vi "vTab_9234_CHx3.vi"() -> ()   [LabVIEW 2018]
uses:
  <vilib>/Utility/sysdir.llb/System Directory Type.ctl
  <vilib>/measure/mamon.llb/Trigger Detection for 1 Channel.vi
  <vilib>/express/express analysis/Spectral/Block/exnSpectralBlock spectral measurements peak poly.vi
  <vilib>/express/express analysis/Spectral/Block/exnSpectralBlock spectral measurements peak DDT.vi
  <vilib>/ErrorRing/Error Ring.xnode
  <vilib>/express/express analysis/Spectral/XNode/ExpressSpectralMeasurementsBlockNode.xnode
  <vilib>/measure/NI_MAPro.lvlib
  <vilib>/Utility/config.llb/NI_LVConfig.lvlib
panel:
  out "SVING":bool caption="存檔"
  in  "Open Folder":bool
  in  "Enable Saving":bool
  in  "Status":bool
  out "DA":bool caption="觸發"
  out "Time":timestamp format="%<%Y/%m/%d   %H:%M:%S>T"
  in  "Tab Control":enum32{"觸發訊號", "參數設定"}(tab)
  out "TD-P2P-Ch 3":dbl
  out "FFT-P2P-Ch 3":dbl
  out "TD-P2P-Ch 2":dbl
  out "FFT-P2P-Ch 2":dbl
  out "TD-P2P-Ch 1":dbl
  out "FFT-P2P-Ch 1":dbl
  out "CH3-Z-FFT":dynamicdata(graph)
  out "CH2-Y-FFT":dynamicdata(graph)
  out "CH1-X-FFT":dynamicdata(graph)
  out "CH3-Z-Timedomain":dynamicdata(graph)
  out "CH2-Y-Timedomain":dynamicdata(graph)
  out "CH1-X-Timedomain":dynamicdata(graph)
  in  "Lower Cut-Off (Hz)":dbl=100.0
  in  "Pre Samples":i32
  in  "Trigger Level":dbl=0.1 format="%#_13g"
  in  "觸發軸":enum32{"Channel 1", "Channel 2", "Channel 3"}(ring)
  in  "DAQ Device (請選取 NI 9234 )":tag="cDAQ1Mod1"
  in  "ABORT":bool
  in  "Run":bool
  out "DAQ Stoped":bool
  out "DAQ Data":dynamicdata(graph)
  in  "PAUSE":bool
  out "DAQ Error":errorcluster
  out "DAQ (N)":i32
  out "Main (N)":i32
  out "Buffer in Queue":i32(slide) scale=0.0..100.0
  out "Processed":dynamicdata(graph)
  in  "Sample Rate":dbl=10000.0 format="%#_13g"
  in  "Samples to Read":i32=10000
  in  "Trigger Slope":enum16{"Falling Edge", "Rising Edge"}(ring)=enum."Rising Edge"
  # "使用前請至 參數設置 設定"
  # "本頁畫面顯示為 觸發後訊號"
  # "FFT Filter by useing High-pass with Lower Cut-Off (Hz)"
  # "擷取卡設定"
  # "(系統開啟後修改無效)"
  # "軟體觸發設定"
  # "(修改即套用)"
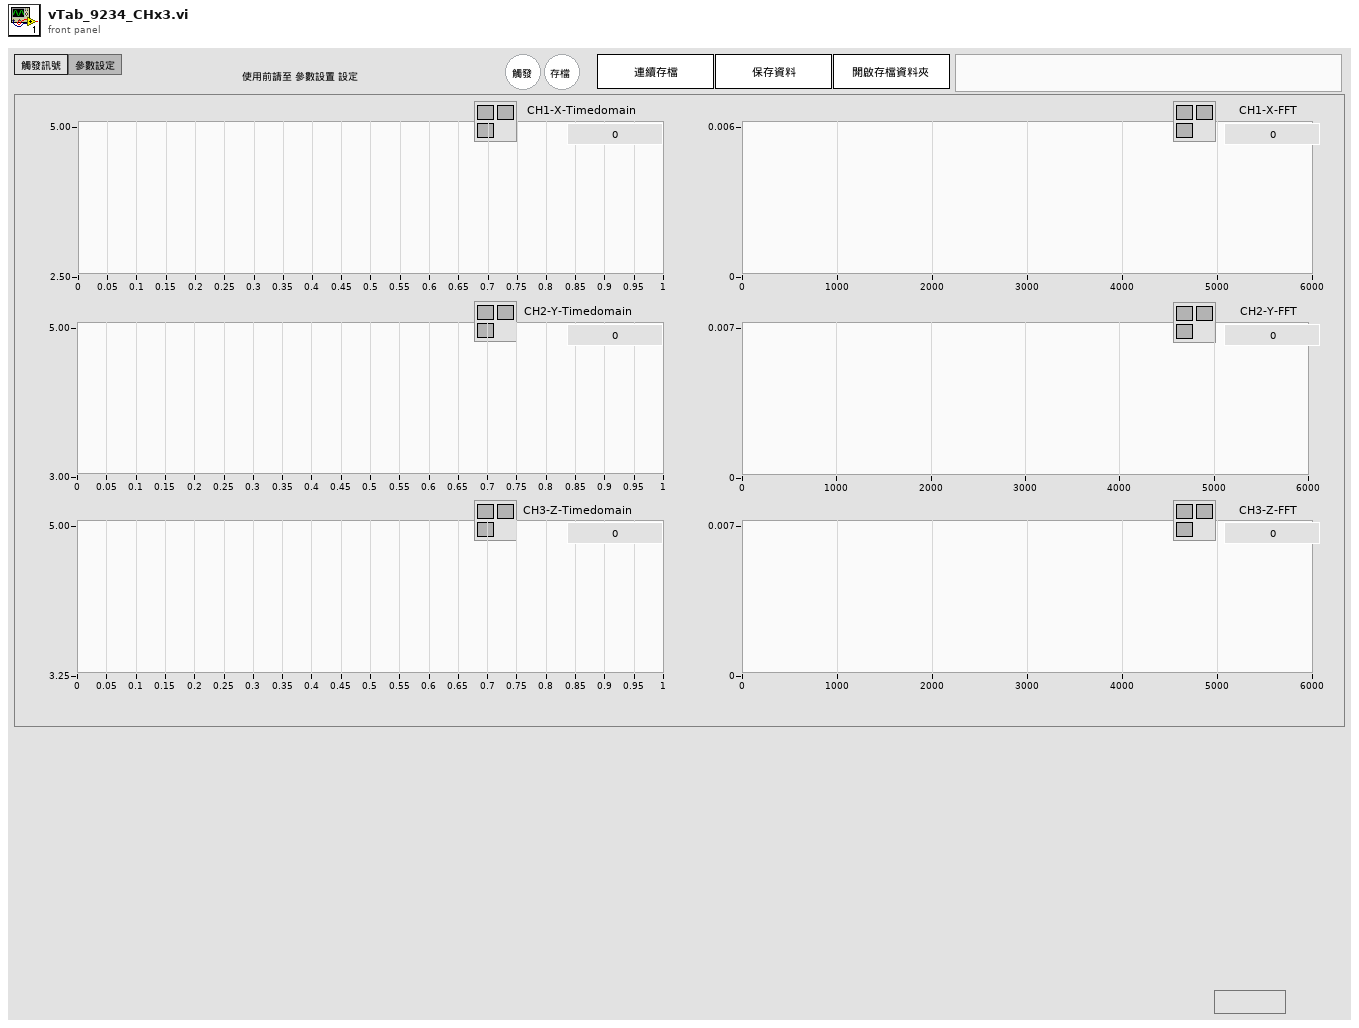
[diagram p1: front panel]
types:
  T1 = typedef "NI_LVConfig.lvlib/Config Data RefNum.ctl" = refnum<k1>
  T2 = enum8{"Enabled", "Disabled", "Disabled and Grayed Out"}
  T3 = cluster{"averaging mode":u16, "weighting mode":u16, "number of averages":u32}
  T4 = cluster{"dB On (F)":bool, "unwrap phase (F)":bool, "convert to degree (F)":bool}
  T5 = typedef "System Directory Type.ctl" = i32
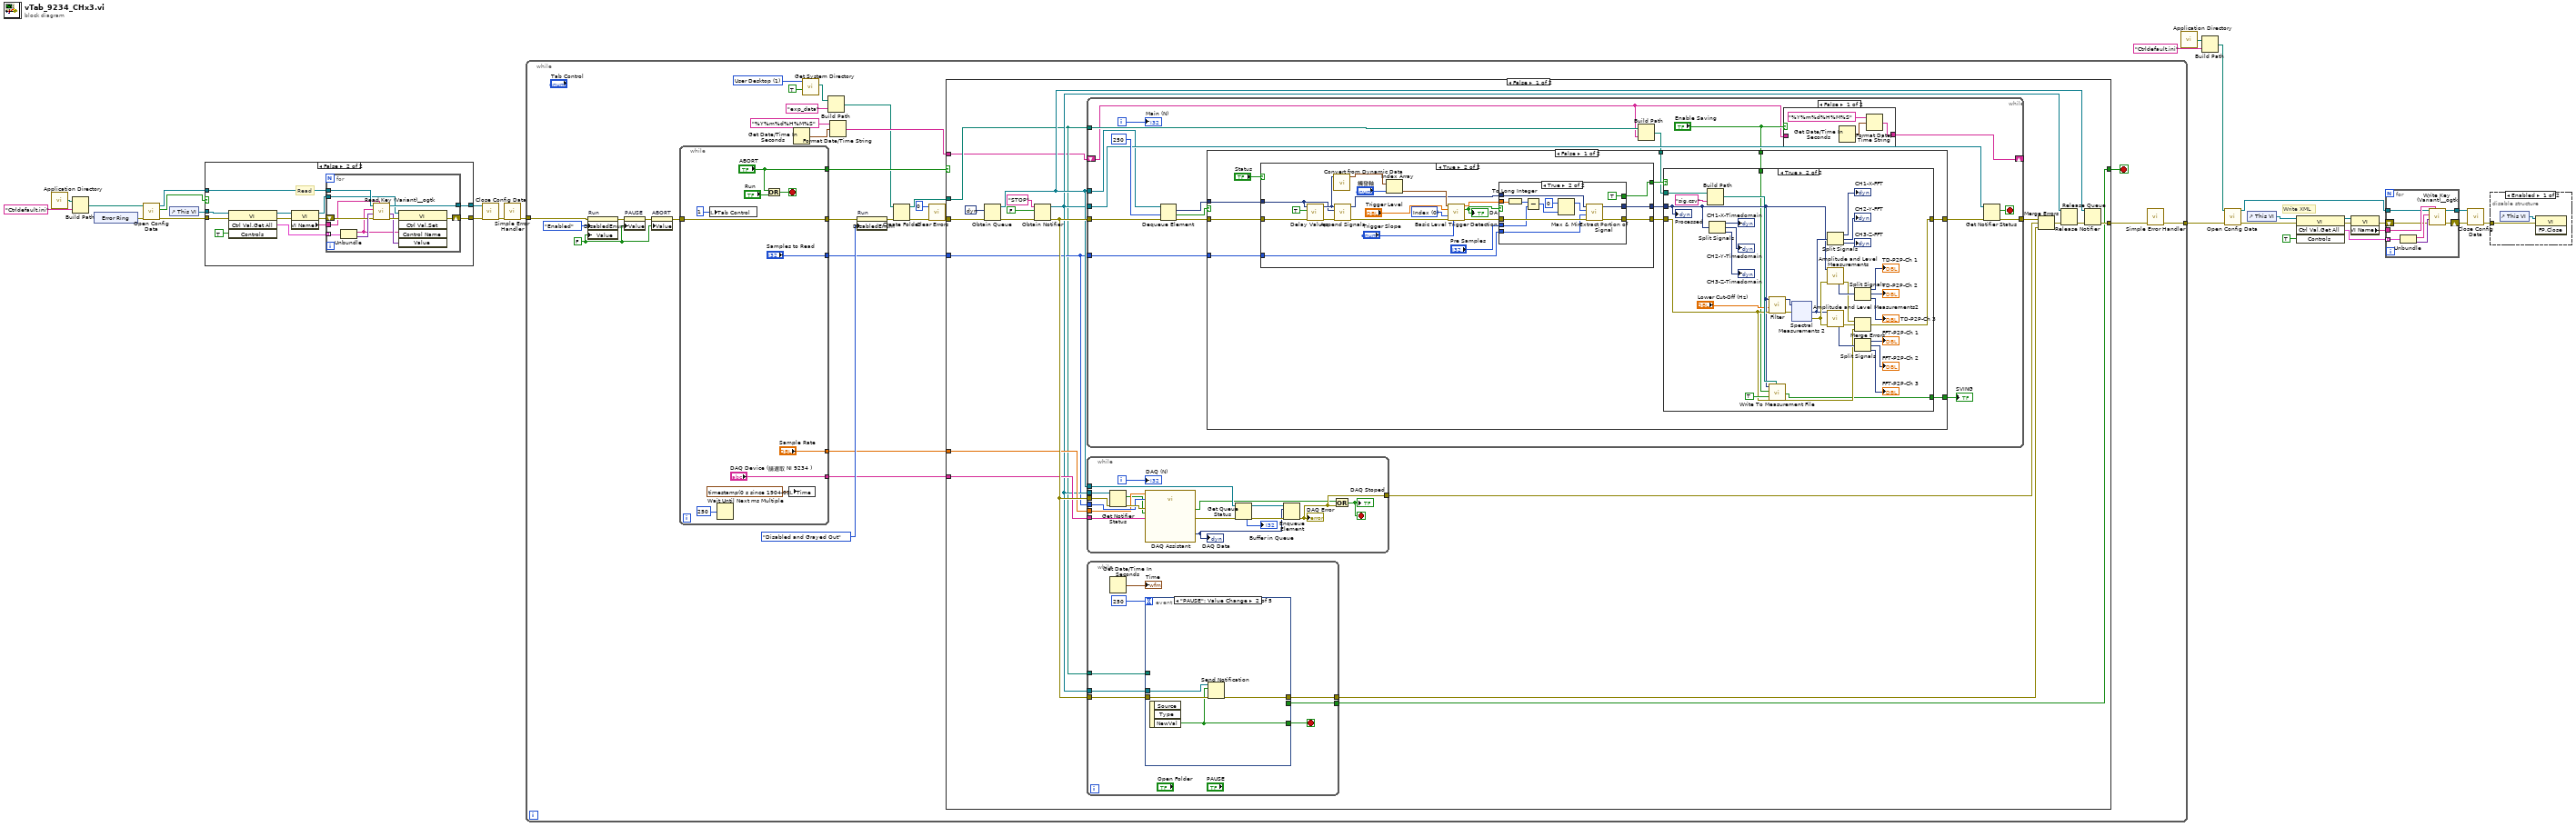
[diagram p0: block diagram]
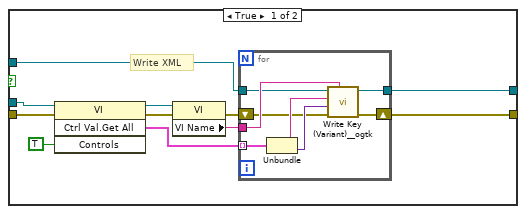
[diagram p2: hidden frame]
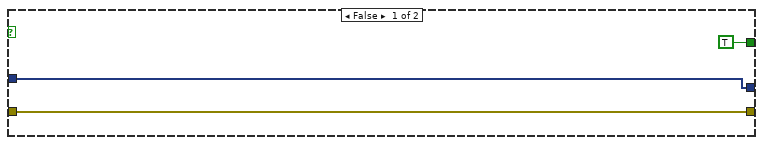
[diagram p5: hidden frame]
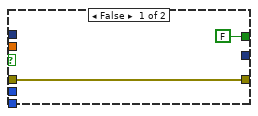
[diagram p6: hidden frame]
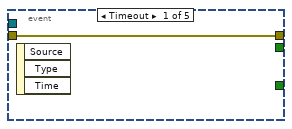
[diagram p9: hidden frame]
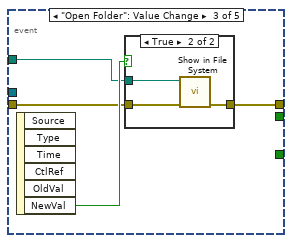
[diagram p10: hidden frame]
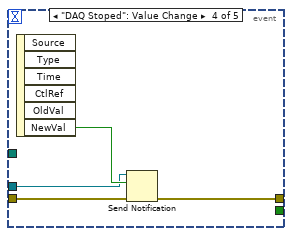
[diagram p12: hidden frame]
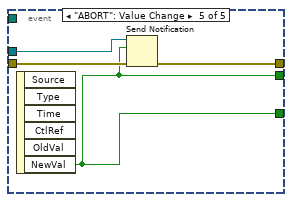
[diagram p13: hidden frame]
diagram:
  # "Write XML"
  n1 = call <vilib>:"Application Directory.vi"() -> ("Application Directory"=w1:path)
  n2 = Build Path(base path=w1, name or relative path="Ctrldefault.ini") -> (appended path=w28:path)
  n3 = xnode "Error Ring"() -> ("error out"=w20:errorcluster)
  n4 = call <vilib>:"Open Config Data.vi"("error in (no error)"=w20, "configuration file path"=w28) -> ("error out"=w25:errorcluster, "file created?"=w21:bool, "refnum"=w18:T1)  [unwired: 7 in]
  n5 = control-ref of="This VI"() -> (w19:refnum<vi>)
  n6 = case shown="False" w21 {
    tunnel: [w33 w53] -> w26
    tunnel: w25 -> [w31 w51]
    tunnel: [w29 w49] -> w24
    tunnel: w19 -> [w32 w52]
    tunnel: w18 -> [w34 w54]
    frame True {
      # "Write XML"
      n7 = invoke class="VI" method="Ctrl Val.Get All"(reference=w32, error in=w31, "Controls"=TRUE) -> (reference out=w38:refnum<vi>, error out=w37:errorcluster, "Get All Control Values Variant"=w39:cluster{"Name":string, "Variant Data":variant}[])  [unwired: 1 in, 1 out]
      n8 = property class="VI"(reference=w38, error in=w37) -> (error out=w30:errorcluster, "VI Name"=w36:string)  [unwired: 1 out]
      n9 = for {
        tunnel: w39 -> [w47] mode=indexing
        tunnel: w36 -> [w46]
        tunnel: w34 -> [w44]
        shift-right: [w43] -> w33
        shift-left: w30 -> [w41]
        tunnel: [w40] -> w29
        n10 = Unbundle(w47) -> ("Name"=w45:string, "Variant Data"=w42:variant)
        n11 = call <userlib>:"Write Key (Variant)__ogtk.vi"("section"=w46, "error in (no error)"=w41, "key-value"=w42, "key (optional)"=w45, "refnum"=w44) -> ("error out"=w43:errorcluster, "refnum out"=w40:T1)  [unwired: 5 in]
      }
    }
    frame False {
      # "Read"
      n12 = invoke class="VI" method="Ctrl Val.Get All"(reference=w52, error in=w51, "Controls"=TRUE) -> (reference out=w58:refnum<vi>, error out=w57:errorcluster, "Get All Control Values Variant"=w59:cluster{"Name":string, "Variant Data":variant}[])  [unwired: 1 in, 1 out]
      n13 = property class="VI"(reference=w58, error in=w57) -> (reference out=w48:refnum<vi>, error out=w50:errorcluster, "VI Name"=w56:string)
      n14 = for {
        tunnel: w59 -> [w70] mode=indexing
        tunnel: w56 -> [w63]
        tunnel: w54 -> [w69]
        shift-right: [w64] -> w53
        shift-left: w50 -> [w67]
        tunnel: [w66] -> w49
        tunnel: w48 -> [w62]
        n15 = Unbundle(w70) -> ("Name"=w60:string, "Variant Data"=w68:variant)
        n16 = call <userlib>:"Read Key (Variant)__ogtk.vi"("section"=w63, "error in (no error)"=w67, "type"=w68, "key (optional)"=w60, "refnum"=w69) -> ("error out"=w65:errorcluster, "key-value"=w61:variant, "refnum out"=w66:T1)  [unwired: 3 in, 1 out]
        n17 = invoke class="VI" method="Ctrl Val.Set"(reference=w62, error in=w65, "Control Name"=w60, "Value"=w61) -> (error out=w64:errorcluster)  [unwired: 1 in, 4 out]
      }
    }
  }
  n18 = call <vilib>:"Close Config Data.vi"("error in (no error)"=w26, "refnum"=w24) -> ("error out"=w23:errorcluster)  [unwired: 8 in, 1 out]
  n19 = call <vilib>:"Simple Error Handler.vi"("error in (no error)"=w23) -> ("error out"=w22:errorcluster)  [unwired: 4 in, 4 out]
  n20 = while {
    tunnel: [w98] -> w4
    tunnel: w22 -> [w76]
    stop <- w79 stop-if-true
    w87 = T5 1 items=["User Home"=0, "User Desktop"=1, "User Documents"=2, "User Application Data"=3, "User Preferences"=4, "User Temporary"=5, "Public Documents"=6, "Public Application Data"=7, "Public Preferences"=8, "Public Cache"=13, "System Core Libraries"=9, "System Installed Libraries"=10, "Application Files"=11, "Boot Volume Root"=12] ("system directory type")
    w92 = FALSE ("stop 3")
    n21 = property on="Run" class="Bool (strict)"(error in=w76, "DisabledEnum"=T2."Enabled" ("Disabled"), "Value"=w92) -> (error out=w95:errorcluster)  [unwired: 1 in, 1 out]
    n22 = property on="PAUSE" class="Bool (strict)"(error in=w95, "Value"=w92) -> (error out=w94:errorcluster)  [unwired: 1 in, 1 out]
    n23 = property on="ABORT" class="Bool (strict)"(error in=w94, "Value"=w92) -> (error out=w93:errorcluster)  [unwired: 1 in, 1 out]
    n24 = while {
      tunnel: [w290] -> w75
      tunnel: w93 -> [w290]
      tunnel: ["Samples to Read"] -> w78
      tunnel: ["Sample Rate"] -> w82
      tunnel: ["DAQ Device (請選取 NI 9234 )"] -> w80
      tunnel: ["ABORT"] -> w74
      stop <- w283 stop-if-true
      n25 = local write "Tab Control"(1) -> ()
      n26 = Wait Until Next ms Multiple(millisecond multiple=u32 250) -> ()  [unwired: 1 out]
      n27 = Or(x="ABORT", y="Run") -> (x .or. y?=w283:bool)
      n28 = local write "Time"(timestamp(0 s since 1904-01-01) ("Time 2")) -> ()
    }
    n29 = Get Date/Time In Seconds() -> (seconds since 1Jan1904=w73:timestamp)
    n30 = call <vilib>:"Get System Directory.vi"("create directory if not found? (F)"=TRUE, "system directory type"=w87) -> ("system directory"=w89:path)  [unwired: 9 in]
    n31 = Build Path(base path=w89, name or relative path="exp_data") -> (appended path=w71:path)
    n32 = Format Date/Time String(time format string (%c)="%Y%m%d%H%M%S", seconds (now)=w73) -> (date/time string=w72:string)  [unwired: 1 in]
    n33 = property on="Run" class="Bool (strict)"(error in=w75, "DisabledEnum"=T2."Disabled and Grayed Out" ("Disabled")) -> (error out=w90:errorcluster)  [unwired: 1 in, 1 out]
    n34 = Create Folder(path (use dialog)=w71, error in=w90) -> (created path=w77:path, error out=w84:errorcluster)  [unwired: 1 in, 1 out]
    n35 = call <vilib>:"Clear Errors.vi"("error in (no error)"=w84, "specific error code to clear (0: all)"=0) -> ("error out"=w83:errorcluster)  [unwired: 4 in, 1 out]
    n36 = case shown="False" w74 {
      selector: w74 -> [_ w279]
      tunnel: w83 -> [w111 w280]
      tunnel: w82 -> [w110 _]
      tunnel: [w107 w280] -> w81
      tunnel: w80 -> [w104 _]
      tunnel: [w102 w279] -> w79
      tunnel: w78 -> [w101 _]
      tunnel: w77 -> [w100 _]
      tunnel: w72 -> [w99 _]
      frame False {
        n37 = Obtain Queue(element data type=dynamicdata [] ("data"), error in (no error)=w111) -> (queue out=w109:refnum<queue>, error out=w114:errorcluster)  [unwired: 3 in, 1 out]
        n38 = Obtain Notifier(name (unnamed)="STOP", notification data type=FALSE, error in (no error)=w114) -> (notifier out=w103:refnum<notifier>, error out=w117:errorcluster)  [unwired: 1 in, 1 out]
        n39 = while {
          tunnel: w109 -> [w127]
          tunnel: w117 -> [w134]
          tunnel: [w130] -> w105
          tunnel: w103 -> [w128]
          tunnel: w101 -> [w125]
          tunnel: w100 -> [w123]
          shift-right: [w120] -> _
          shift-left: w99 -> [w119]
          i -> [w136]
          stop <- w129 stop-if-true
          n40 = Dequeue Element(queue=w127, timeout in ms (-1)=250, error in (no error)=w134) -> (element=w133:dynamicdata, timed out?=w126:bool, error out=w132:errorcluster)  [unwired: 1 out]
          n41 = Build Path(base path=w123, name or relative path=w119) -> (appended path=w122:path)
          n42 = case shown="False" w126 {
            tunnel: w133 -> [w150 _]
            tunnel: w132 -> [w148 w232]
            tunnel: [w151 w232] -> w131
            tunnel: w125 -> [w144 _]
            tunnel: w122 -> [w143 _]
            tunnel: [w142 _] -> w124
            tunnel: "Enable Saving" -> [w141 _]
            frame False {
              n43 = case shown="True" "Status" {
                tunnel: [TRUE ("Data Available") w159] -> w145
                tunnel: w150 -> [w154 w164]
                tunnel: [w154 w157] -> w149
                tunnel: w148 -> [w153 w166]
                tunnel: [w153 w158] -> w147
                tunnel: w144 -> [_ w155]
                frame False {
                }
                frame True {
                  w171 = u16 0 items=["Index", "Time"] ("location mode")
                  n44 = call "Delay Values"("error in (no error)"=w166, "Enable"=TRUE, "Signals"=w164) -> ("error out"=w163:errorcluster, "Delayed Signals"=w165:dynamicdata)  [unwired: 7 in]
                  n45 = call "Convert from Dynamic Data"("Dynamic Data Type"=w165) -> ("Array of Waveform"=w175:waveform(dbl)[])  [unwired: 3 in]
                  n46 = call "Append Signals"("error in (no error)"=w163, "Input Signal B"=w164, "Input Signal A"=w165) -> ("error out"=w162:errorcluster, "Appended Signals"=w160:dynamicdata)  [unwired: 7 in]
                  n47 = Index Array(array=w175, index="觸發軸") -> (element=w174:waveform(dbl))
                  n48 = call-poly <vilib>:"Basic Level Trigger Detection.vi"("signal in"=w174, "level"="Trigger Level", "location mode"=w171, "error in (no error)"=w162, "trigger slope"="Trigger Slope") -> ("trigger location"=w168:dbl, "trigger detected?"=w169:bool, "error out"=w161:errorcluster)  [unwired: 8 in]
                  "DA" <- w169
                  n49 = case shown="True" w169 {
                    tunnel: w168 -> [_ w188]
                    tunnel: w161 -> [w176 w189]
                    tunnel: w160 -> [_ w183]
                    tunnel: [FALSE ("Enable") TRUE ("Enable")] -> w159
                    tunnel: [w176 w186] -> w158
                    tunnel: [_ w184] -> w157
                    tunnel: "Pre Samples" -> [_ w181]
                    tunnel: w155 -> [_ w178]
                    frame False {
                    }
                    frame True {
                      n50 = To Long Integer(number=w188) -> (32bit integer=w187:i32)
                      n51 = Subtract(x=w187, y=w181) -> (x-y=w182:i32)
                      n52 = Max & Min(x=0, y=w182) -> (max(x,y)=w179:i32)  [unwired: 1 out]
                      n53 = call "Extract Portion of Signal"("error in (no error)"=w189, "Samples"=w178, "Begin Sample"=w179, "Signals"=w183) -> ("error out"=w186:errorcluster, "Section"=w184:dynamicdata)  [unwired: 6 in]
                    }
                  }
                }
              }
              n54 = case shown="True" w145 {
                tunnel: w149 -> [_ w195]
                tunnel: w147 -> [w190 w197]
                tunnel: [w190 w203] -> w151
                tunnel: w143 -> [_ w201]
                tunnel: [_ w192] -> w142
                tunnel: w141 -> [_ w191]
                frame False {
                }
                frame True {
                  n55 = Build Path(base path=w201, name or relative path="sig.csv") -> (appended path=w199:path)
                  n56 = Split Signals(w195) -> (→"CH1-X-Timedomain":dynamicdata, →"CH2-Y-Timedomain":dynamicdata, →"CH3-Z-Timedomain":dynamicdata)  [unwired: 3 in]
                  n57 = call "Filter"("error in (no error)"=w197, "Lower Cut-Off"="Lower Cut-Off (Hz)", "Signal"=w195) -> ("error out"=w196:errorcluster, "Filtered Signal"=w194:dynamicdata)  [unwired: 7 in]
                  n58 = call "Write To Measurement File"("Signals"=w195, "Enable"=w191, "new_file"=TRUE, "error in (no error)"=w197, "Filename"=w199) -> ("Saving Data"=w192:bool, "error out"=w206:errorcluster)  [unwired: 12 in, 1 out]
                  n59 = xnode ("Spectral Measurements 2")("Signals"=w194, "error in (no error)"=w196) -> ("FFT - (Peak)"=w198:dynamicdata, "error out"=w221:errorcluster)  [unwired: 1 out]
                  n60 = Split Signals(w198) -> (→"CH1-X-FFT":dynamicdata, →"CH2-Y-FFT":dynamicdata, →"CH3-Z-FFT":dynamicdata)  [unwired: 3 in]
                  n61 = call "Amplitude and Level Measurements"("Signals"=w195, "error in (no error)"=w221) -> ("Peak to Peak"=w208:dynamicdata, "error out"=w204:errorcluster)  [unwired: 12 out]
                  n62 = call "Amplitude and Level Measurements2"("Signals"=w198, "error in (no error)"=w221) -> ("Peak to Peak"=w207:dynamicdata, "error out"=w205:errorcluster)  [unwired: 12 out]
                  n63 = Split Signals(w208) -> (→"TD-P2P-Ch 1":dynamicdata, →"TD-P2P-Ch 2":dynamicdata, →"TD-P2P-Ch 3":dynamicdata)  [unwired: 3 in]
                  n64 = Merge Errors(w204, w205, w206) -> (w203:errorcluster)
                  n65 = Split Signals(w207) -> (→"FFT-P2P-Ch 1":dynamicdata, →"FFT-P2P-Ch 2":dynamicdata, →"FFT-P2P-Ch 3":dynamicdata)  [unwired: 3 in]
                  "Processed" <- w195
                }
              }
            }
            frame True {
            }
          }
          "SVING" <- w124
          n66 = case shown="False" "Enable Saving" {
            tunnel: [w137 w140] -> w120
            tunnel: w119 -> [_ w140]
            frame False {
              n67 = Get Date/Time In Seconds() -> (seconds since 1Jan1904=w138:timestamp)
              n68 = Format Date/Time String(time format string (%c)="%Y%m%d%H%M%S", seconds (now)=w138) -> (date/time string=w137:string)  [unwired: 1 in]
            }
            frame True {
            }
          }
          n69 = Get Notifier Status(notifier=w128, error in (no error)=w131) -> (current notification=w129:bool, error out=w130:errorcluster)  [unwired: 3 out]
          "Main (N)" <- w136
        }
        n70 = while {
          tunnel: w109 -> [w247]
          tunnel: [w239] -> w116
          tunnel: w117 -> [w243]
          tunnel: w103 -> [w241]
          tunnel: w101 -> [w238]
          tunnel: w110 -> [w237]
          tunnel: w104 -> [w233]
          i -> [w249]
          stop <- w240 stop-if-true
          n71 = Get Notifier Status(notifier=w241, error in (no error)=w243) -> (current notification=w236:bool, error out=w242:errorcluster)  [unwired: 3 out]
          n72 = call "DAQ Assistant"("rate"=w237, "number of samples"=w238, "error in"=w242, "stop (F)"=w236, "device name"=w233) -> ("data"=w234:dynamicdata, "stopped"=w235:bool, "error out"=w244:errorcluster)  [unwired: 11 in, 1 out]
          "DAQ Data" <- w234
          n73 = Get Queue Status(queue=w247, error in (no error)=w244) -> (queue out=w246:refnum<queue>, error out=w245:errorcluster, # elements in queue=→"Buffer in Queue":i32)  [unwired: 1 in, 5 out]
          n74 = Enqueue Element(queue=w246, element=w234, error in (no error)=w245) -> (error out=w239:errorcluster)  [unwired: 1 in, 2 out]
          "DAQ Error" <- w239
          n75 = Compound Arithmetic op=OR(w235, w239) -> (w240:bool)
          "DAQ Stoped" <- w240
          "DAQ (N)" <- w249
        }
        n76 = while {
          tunnel: w117 -> [w257]
          tunnel: [w256] -> w118
          tunnel: w103 -> [w254]
          tunnel: [w251] -> w102
          tunnel: w100 -> [w250]
          stop <- w252 stop-if-true
          n77 = Get Date/Time In Seconds() -> (seconds since 1Jan1904=→"Time":timestamp)
          n78 = event shown="[1] \"PAUSE\": Value Change" {
            selector: _ -> [_ _ _ _ _]
            dyn-events: _ -> [_ _ _ _ _]
            timeout: 250 -> [_ _ _ _ _]
            tunnel: w257 -> [w258 w262 w265 w274 w278]
            tunnel: [w258 w261 w263 w271 w277] -> w256
            tunnel: w254 -> [_ w260 _ w272 w276]
            tunnel: [_ w259 _ _ w275] -> w252
            tunnel: [_ _ _ _ w275] -> w251
            tunnel: w250 -> [_ _ w264 _ _]
            event Timeout {
              n79 = event-data() -> ()  [unwired: 1 in, 3 out]
            }
            event "PAUSE": Value Change {
              n80 = event-data() -> ("NewVal"=w259:bool)  [unwired: 1 in, 2 out]
              n81 = Send Notification(notification=w259, notifier=w260, error in (no error)=w262) -> (error out=w261:errorcluster)  [unwired: 1 out]
            }
            event "Open Folder": Value Change {
              n82 = event-data() -> ("NewVal"=w266:bool)  [unwired: 1 in, 5 out]
              n83 = case shown="True" w266 {
                tunnel: w265 -> [w267 w270]
                tunnel: w264 -> [_ w269]
                tunnel: [w267 w268] -> w263
                frame False {
                }
                frame True {
                  n84 = call <vilib>:"Show in File System.vi"("error in (no error)"=w270, "file or directory path"=w269) -> ("error out"=w268:errorcluster)  [unwired: 9 in]
                }
              }
            }
            event "DAQ Stoped": Value Change {
              n85 = event-data() -> ("NewVal"=w273:bool)  [unwired: 1 in, 5 out]
              n86 = Send Notification(notification=w273, notifier=w272, error in (no error)=w274) -> (error out=w271:errorcluster)  [unwired: 1 out]
            }
            event "ABORT": Value Change {
              n87 = event-data() -> ("NewVal"=w275:bool)  [unwired: 1 in, 5 out]
              n88 = Send Notification(notification=w275, notifier=w276, error in (no error)=w278) -> (error out=w277:errorcluster)  [unwired: 1 out]
            }
          }
        }
        n89 = Merge Errors(w105, w116, w118) -> (w106:errorcluster)
        n90 = Release Notifier(notifier=w103, error in (no error)=w106) -> (error out=w108:errorcluster)  [unwired: 1 in, 2 out]
        n91 = Release Queue(queue=w109, error in (no error)=w108) -> (error out=w107:errorcluster)  [unwired: 1 in, 2 out]
      }
      frame True {
      }
    }
    n92 = call <vilib>:"Simple Error Handler.vi"("error in (no error)"=w81) -> ("error out"=w98:errorcluster)  [unwired: 4 in, 4 out]
  }
  n93 = call <vilib>:"Application Directory.vi"() -> ("Application Directory"=w2:path)
  n94 = Build Path(base path=w2, name or relative path="Ctrldefault.ini") -> (appended path=w11:path)
  n95 = call <vilib>:"Open Config Data.vi"("error in (no error)"=w4, "configuration file path"=w11) -> ("error out"=w14:errorcluster, "refnum"=w17:T1)  [unwired: 7 in, 1 out]
  n96 = control-ref of="This VI"() -> (w16:refnum<vi>)
  n97 = invoke class="VI" method="Ctrl Val.Get All"(reference=w16, error in=w14, "Controls"=TRUE) -> (reference out=w9:refnum<vi>, error out=w8:errorcluster, "Get All Control Values Variant"=w10:cluster{"Name":string, "Variant Data":variant}[])  [unwired: 1 in, 1 out]
  n98 = property class="VI"(reference=w9, error in=w8) -> (error out=w5:errorcluster, "VI Name"=w7:string)  [unwired: 1 out]
  n99 = for {
    tunnel: w10 -> [w298] mode=indexing
    tunnel: w7 -> [w297]
    tunnel: w17 -> [w295]
    shift-right: [w294] -> w13
    shift-left: w5 -> [w292]
    tunnel: [w291] -> w15
    n100 = Unbundle(w298) -> ("Name"=w296:string, "Variant Data"=w293:variant)
    n101 = call <userlib>:"Write Key (Variant)__ogtk.vi"("section"=w297, "error in (no error)"=w292, "key-value"=w293, "key (optional)"=w296, "refnum"=w295) -> ("error out"=w294:errorcluster, "refnum out"=w291:T1)  [unwired: 5 in]
  }
  n102 = call <vilib>:"Close Config Data.vi"("error in (no error)"=w13, "refnum"=w15) -> ("error out"=w3:errorcluster)  [unwired: 8 in, 1 out]
  n103 = disable-structure shown="Enabled" {
    disable-tunnel: w3 -> [w299 _]
    frame Enabled {
      n104 = control-ref of="This VI"() -> (w300:refnum<vi>)
      n105 = invoke class="VI" method="FP.Close"(reference=w300, error in=w299) -> ()  [unwired: 1 in, 3 out]
    }
    frame Disabled {
    }
  }
